vi "GMonitor.vi"(5 "Time Stamp":timestamp, 6 "v1":dbl[](array[numeric]), 7 "v0":dbl[](array[numeric]), 8 "lockin information":T1, 9 "tdms file":refnum<k34>) -> (0 "FtR":dbl, 1 "FtG":dbl, 2 "TtR":dbl, 3 "TtG":dbl, 4 "tdms file out":refnum<k34>)   [LabVIEW 2013]
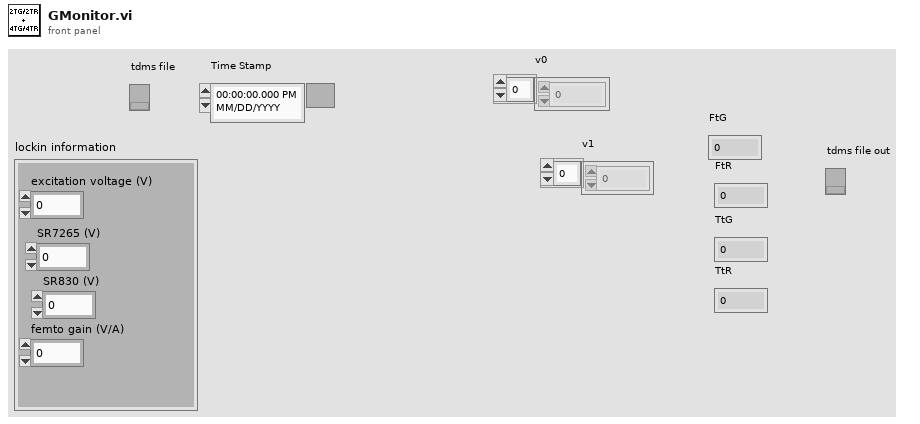
[diagram p1: front panel]
types:
  T1 = cluster{"excitation voltage (V)":dbl, "SR7265 (V)":dbl, "SR830 (V)":dbl, "femto gain (V/A)":dbl}
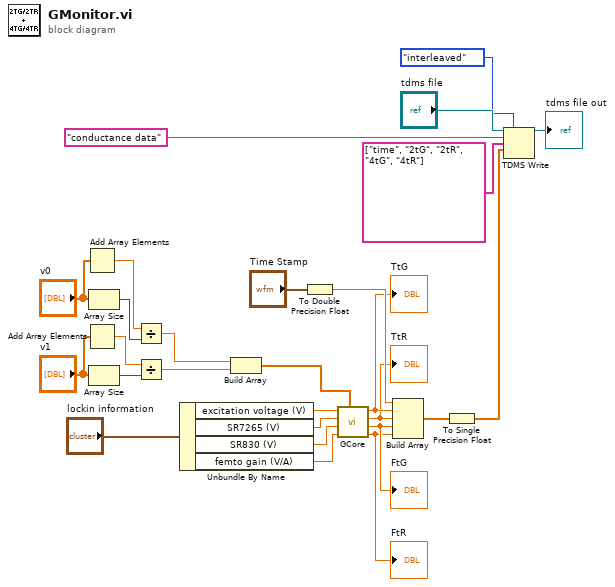
[diagram p0: block diagram]
diagram:
  n1 = Add Array Elements(numeric array="v0") -> (sum=w26:dbl)
  n2 = Add Array Elements(numeric array="v1") -> (sum=w23:dbl)
  n3 = Array Size(array="v0") -> (size(s)=w25:i32)
  n4 = Array Size(array="v1") -> (size(s)=w22:i32)
  n5 = Divide(x=w26, y=w25) -> (x/y=w12:dbl)
  n6 = Divide(x=w23, y=w22) -> (x/y=w11:dbl)
  n7 = Unbundle By Name("lockin information") -> ("excitation voltage (V)"=w8:dbl, "SR7265 (V)"=w7:dbl, "SR830 (V)"=w6:dbl, "femto gain (V/A)"=w5:dbl)
  n8 = Build Array(w12, w11) -> (w10:dbl[])
  n9 = To Double Precision Float(number="Time Stamp") -> (double precision float=w20:dbl)
  n10 = call "GCore.vi"("G data"=w10, "Femto Gain (V/A)"=w5, "SR830 sensitivity"=w6, "SR7265 sensitivity (V)"=w7, "Excitation voltage (V)"=w8) -> ("4tR"=w1:dbl, "4tG"=w2:dbl, "2tR"=w3:dbl, "2tG"=w4:dbl)
  "TtG" <- w4
  "TtR" <- w3
  "FtG" <- w2
  "FtR" <- w1
  n11 = Build Array(w20, w4, w3, w2, w1) -> (w17:dbl[])
  n12 = To Single Precision Float(number=w17) -> (single precision float=w16:sgl[])
  n13 = TDMS Write(0:"tdms file", 1:enum16{"decimated", "interleaved"}."interleaved" ("data layout (0:decimated)"), 5:"conductance data", 7:string[] ["time", "2tG", "2tR", "4tG", "4tR"], 9:w16) -> (4:→"tdms file out":refnum<k34>)  [unwired: 1 in, 3 out]
